vi "SRV_Match String in Array of Patterns.vi"(0 "string":string, 7 "regular expressions":string[](array[string])) -> (4 "before substring":string, 6 "match substring":string, 8 "after substring":string, 10 "offset past match":i32, 14 "Any Matches?":bool, 15 "index of Match":i32)   [LabVIEW 2014]
doc: "Returns TRUE if any of the patterns in \"regular expressions\" array matches the string. The index of the first matching reg exp is returned.\n\nReturns FALSE and \"-1\" if no matches.\n\n\nAuthor: Mike Schultz - Logic PD"
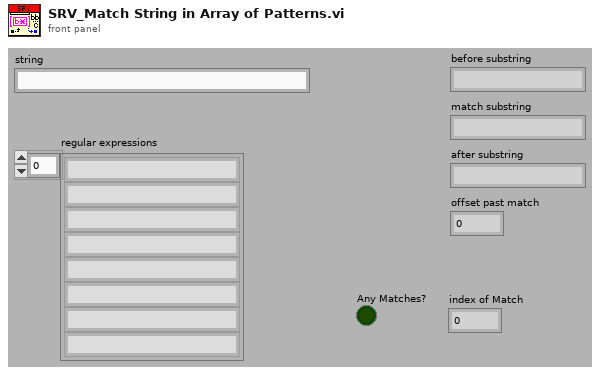
[diagram p1: front panel]
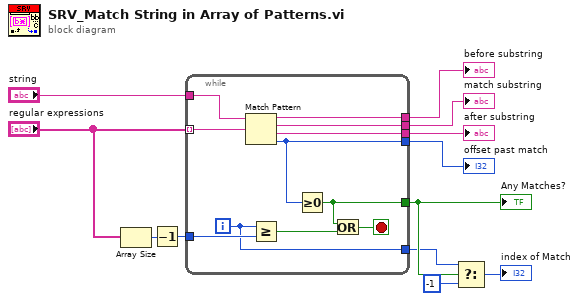
[diagram p0: block diagram]
diagram:
  n1 = Array Size(array="regular expressions") -> (size(s)=w10:i32)
  n2 = Decrement(x=w10) -> (x-1=w9:i32)
  n3 = while {
    tunnel: "regular expressions" -> [w23] mode=indexing
    tunnel: "string" -> [w22]
    tunnel: w9 -> [w20]
    tunnel: [w18] -> w8
    tunnel: [w17] -> w7
    tunnel: [w16] -> w4
    tunnel: [w15] -> w3
    tunnel: [w14] -> w2
    tunnel: [w13] -> w1
    i -> [w17]
    stop <- w21 stop-if-true
    n4 = Match Pattern(string=w22, regular expression=w23) -> (before substring=w16:string, match substring=w15:string, after substring=w14:string, offset past match=w13:i32)  [unwired: 1 out]
    n5 = Greater Or Equal?(x=w17, y=w20) -> (x >= y?=w19:bool)
    n6 = Greater Or Equal To 0?(x=w13) -> (x >= 0?=w18:bool)
    n7 = Or(x=w18, y=w19) -> (x .or. y?=w21:bool)
  }
  "Any Matches?" <- w8
  "before substring" <- w4
  "match substring" <- w3
  "after substring" <- w2
  "offset past match" <- w1
  n8 = Select(t=w7, s=w8, f=-1) -> (s? t:f=→"index of Match":i32)
